vi "BasicExampleHost.vi"() -> ()   [LabVIEW 2015]
uses:
  Interface/Configuration.ctl
  Core/SingleAIConfig.ctl
  <vilib>/FPGAPlugInAG/sbRIO-9607/niLvFpga_Open_sbRIO-9607.vi
  <vilib>/rvi/interface/common/dynamic/niFpgaDynamicAddResources.vi
  <vilib>/Utility/error.llb/Error Cluster From Error Code.vi
  <vilib>/RVI Host/nirviSupport.llb/nirviErrorClusterFromErrorCode.vi
  <vilib>/rvi/errors/niLvFpgaAdjustHostInterfaceError.vi
  <vilib>/FPGAPlugInAG/Dynamic/niLvFpga_Close_Dynamic.vi
  <vilib>/rvi/interface/nirviOpenFPGA/nirviOpenFPGA.xnode
  FPGA Bitfiles/ScaleAndLimit_FPGATarget_BasicFPGATest_5eEjrSJq-IM.lvbitx
  BasicFPGATest.vi
  <vilib>/rvi/interface/nirviMethod/nirviMethod.xnode
  <vilib>/rvi/interface/nirviReadWriteControl/nirviReadWriteControl.xnode
  <vilib>/rvi/interface/nirviCloseFPGA/nirviCloseFPGA.xnode
  Interface/ScaleAndLimitInterface.lvlib
  <vilib>/rvi/interface/Simulation/niFpgaSimulationCallBeginRW.vi
  Core/ScaleAndLimit.lvlib
  <vilib>/rvi/interface/nirviMethod/StockFPGA_InlinedMethodWaitForSingleIRQ.vi
  <vilib>/FPGAPlugInAG/Dynamic/niLvFpga_WaitOnIrq_Dynamic.vi
  <vilib>/FPGAPlugInAG/Dynamic/niLvFpga_AcknowledgeIrq_Dynamic.vi
  NiFpgaLv.dll
panel:
  out "LimitsFlag":bool
  out "LowLimits":u16
  out "HighLimits":u16
  out "UnscaledAI":i16[](array[numeric])
  in  "DummyAI15":i16
  in  "stop":bool
  out "ScaledAI":sgl[](array[numeric])
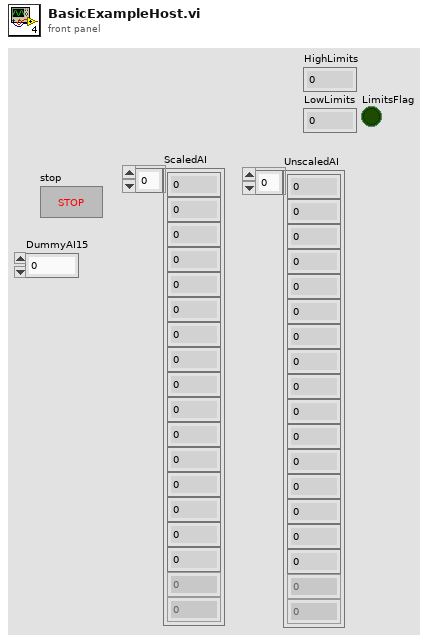
[diagram p1: front panel]
types:
  T1 = typedef "ScaleAndLimitInterface.lvlib/Configuration.ctl" = cluster{"Name":string, "M":dbl, "B":i16, "HighLimit":dbl, "LowLimit":dbl, "LimitsEnabled":bool}
  T2 = typedef "ScaleAndLimit.lvlib/SingleAIConfig.ctl" = cluster{"LimitsEnable":bool, "UnscaledHighLimit":i16, "UnscaledLowLimit":i16, "B":i16, "M":sgl}
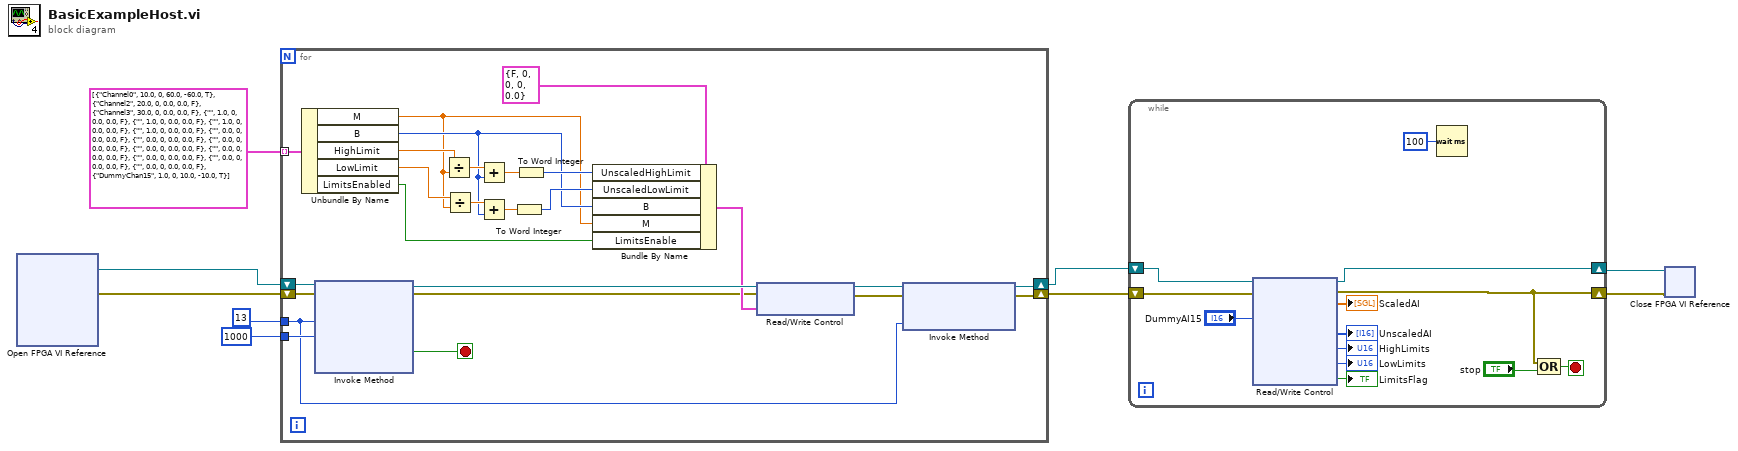
[diagram p0: block diagram]
diagram:
  n1 = xnode "Open FPGA VI Reference"() -> ("FPGA VI Reference Out"=w4:refnum<k20>, "error out"=w5:errorcluster)  [unwired: 2 in]
  n2 = for {
    tunnel: 13 ("IRQ Number") -> [w13]
    tunnel: 1000 ("Timeout (ms)") -> [w33]
    tunnel: T1[] [{"Name"="Channel0", "M"=10.0, "B"=0, "HighLimit"=60.0, "LowLimit"=-60.0, "LimitsEnabled"=TRUE}, {"Name"="Channel2", "M"=20.0, "B"=0, "HighLimit"=0.0, "LowLimit"=0.0, "LimitsEnabled"=FALSE}, {"Name"="Channel3", "M"=30.0, "B"=0, "HighLimit"=0.0, "LowLimit"=0.0, "LimitsEnabled"=FALSE}, {"Name"="", "M"=1.0, "B"=0, "HighLimit"=0.0, "LowLimit"=0.0, "LimitsEnabled"=FALSE}, {"Name"="", "M"=1.0, "B"=0, "HighLimit"=0.0, "LowLimit"=0.0, "LimitsEnabled"=FALSE}, {"Name"="", "M"=1.0, "B"=0, "HighLimit"=0.0, "LowLimit"=0.0, "LimitsEnabled"=FALSE}, {"Name"="", "M"=1.0, "B"=0, "HighLimit"=0.0, "LowLimit"=0.0, "LimitsEnabled"=FALSE}, {"Name"="", "M"=0.0, "B"=0, "HighLimit"=0.0, "LowLimit"=0.0, "LimitsEnabled"=FALSE}, {"Name"="", "M"=0.0, "B"=0, "HighLimit"=0.0, "LowLimit"=0.0, "LimitsEnabled"=FALSE}, {"Name"="", "M"=0.0, "B"=0, "HighLimit"=0.0, "LowLimit"=0.0, "LimitsEnabled"=FALSE}, {"Name"="", "M"=0.0, "B"=0, "HighLimit"=0.0, "LowLimit"=0.0, "LimitsEnabled"=FALSE}, {"Name"="", "M"=0.0, "B"=0, "HighLimit"=0.0, "LowLimit"=0.0, "LimitsEnabled"=FALSE}, {"Name"="", "M"=0.0, "B"=0, "HighLimit"=0.0, "LowLimit"=0.0, "LimitsEnabled"=FALSE}, {"Name"="", "M"=0.0, "B"=0, "HighLimit"=0.0, "LowLimit"=0.0, "LimitsEnabled"=FALSE}, {"Name"="", "M"=0.0, "B"=0, "HighLimit"=0.0, "LowLimit"=0.0, "LimitsEnabled"=FALSE}, {"Name"="DummyChan15", "M"=1.0, "B"=0, "HighLimit"=10.0, "LowLimit"=-10.0, "LimitsEnabled"=TRUE}] ("Configuration") -> [w30] mode=indexing
    shift-right: [w11] -> w7
    shift-left: w5 -> [w32]
    shift-right: [w12] -> w6
    shift-left: w4 -> [w34]
    stop <- w31 stop-if-true
    n3 = Unbundle By Name(w30) -> ("M"=w19:dbl, "B"=w20:i16, "HighLimit"=w29:dbl, "LowLimit"=w28:dbl, "LimitsEnabled"=w18:bool)
    n4 = xnode "Invoke Method"("FPGA VI Reference In"=w34, "error in"=w32, "IRQ Number(s)"=w13, "Timeout (ms)"=w33) -> ("FPGA VI Reference Out"=w17:refnum<k20>, "error out"=w15:errorcluster, "Timed Out"=w31:bool)  [unwired: 1 out]
    n5 = Divide(x=w29, y=w19) -> (x/y=w26:dbl)
    n6 = Divide(x=w28, y=w19) -> (x/y=w27:dbl)
    n7 = Add(x=w26, y=w20) -> (x+y=w25:dbl)
    n8 = Add(x=w27, y=w20) -> (x+y=w24:dbl)
    n9 = To Word Integer(number=w24) -> (16bit integer=w21:i16)
    n10 = To Word Integer(number=w25) -> (16bit integer=w22:i16)
    n11 = Bundle By Name(cluster=T2 {"LimitsEnable"=FALSE, "UnscaledHighLimit"=0, "UnscaledLowLimit"=0, "B"=0, "M"=0.0} ("SingleRawAIConfig"), "UnscaledHighLimit"=w22, "UnscaledLowLimit"=w21, "B"=w20, "M"=w19, "LimitsEnable"=w18) -> (w16:T2)
    n12 = xnode "Read/Write Control"("FPGA VI Reference In"=w17, "error in"=w15, "SingleAIConfig"=w16) -> ("FPGA VI Reference Out"=w14:refnum<k20>, "error out"=w10:errorcluster)
    n13 = xnode "Invoke Method"("FPGA VI Reference In"=w14, "error in"=w10, "IRQ Number(s)"=w13) -> ("FPGA VI Reference Out"=w12:refnum<k20>, "error out"=w11:errorcluster)
  }
  n14 = while {
    shift-right: [w35] -> w1
    shift-left: w6 -> [w46]
    shift-right: [w39] -> w2
    shift-left: w7 -> [w47]
    stop <- w41 stop-if-true
    n15 = xnode "Read/Write Control"("FPGA VI Reference In"=w46, "error in"=w47, "DummyAI15"="DummyAI15") -> ("FPGA VI Reference Out"=w35:refnum<k20>, "error out"=w39:errorcluster, "ScaledAI"=→"ScaledAI":sgl[], "UnscaledAI"=→"UnscaledAI":i16[], "HighLimits"=→"HighLimits":u16, "LowLimits"=→"LowLimits":u16, "LimitsFlag"=→"LimitsFlag":bool)
    n16 = Wait (ms)(milliseconds to wait=u32 100) -> ()  [unwired: 1 out]
    n17 = Compound Arithmetic op=OR(w39, "stop") -> (w41:bool)
  }
  n18 = xnode "Close FPGA VI Reference"("FPGA VI Reference In"=w1, "error in"=w2) -> ()  [unwired: 1 out]
